vi "FileController.vi"() -> ()   [LabVIEW 2018]
panel:
  in  "Overdrive":bool
  in  "New file":bool
  in  "Pause DAQ":bool
  in  "Record":bool
  in  "Valve Log Name":string
  in  "Load Cell Log Name":string
  in  "Sensor Log Name":string
  in  "Log Folder":path
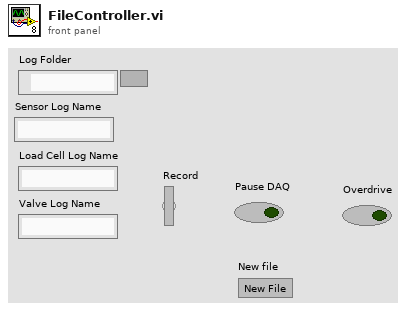
[diagram p1: front panel]
types:
  T1 = cluster{"SensorRecState":refnum<notifier>, "LoadCellRecState":refnum<notifier>, "ValveRecState":refnum<notifier>}
  T2 = enum16{"Normal", "Overdrive", "Ready for Overdrive End", "Ready for new file", "New file"}
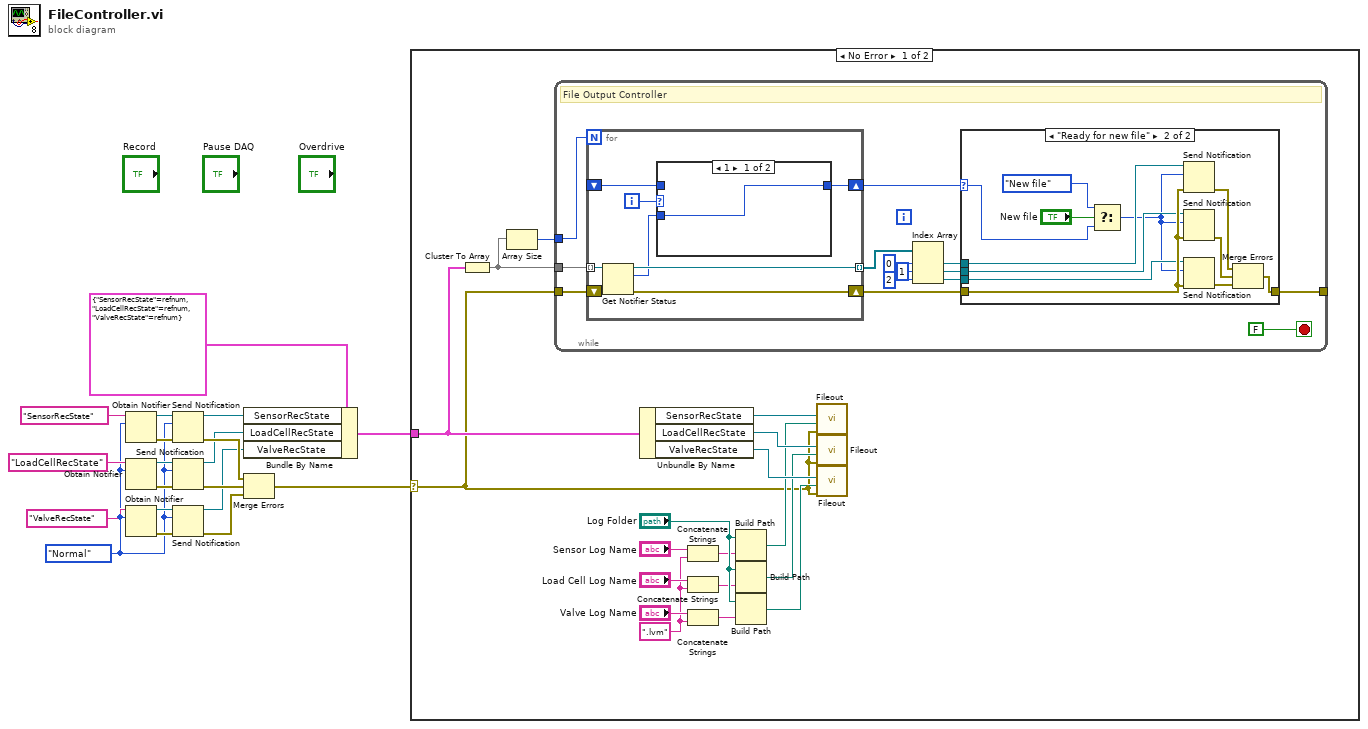
[diagram p0: block diagram]
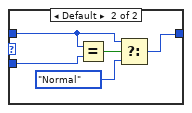
[diagram p3: hidden frame]
diagram:
  w1 = T2."Normal" ("RecState")
  n1 = Obtain Notifier(name (unnamed)="SensorRecState", notification data type=w1) -> (notifier out=w8:refnum<notifier>, error out=w9:errorcluster)  [unwired: 2 in, 1 out]
  n2 = Obtain Notifier(name (unnamed)="LoadCellRecState", notification data type=w1) -> (notifier out=w10:refnum<notifier>, error out=w11:errorcluster)  [unwired: 2 in, 1 out]
  n3 = Obtain Notifier(name (unnamed)="ValveRecState", notification data type=w1) -> (notifier out=w12:refnum<notifier>, error out=w13:errorcluster)  [unwired: 2 in, 1 out]
  n4 = Send Notification(notification=w1, notifier=w8, error in (no error)=w9) -> (notifier out=w7:refnum<notifier>, error out=w6:errorcluster)
  n5 = Send Notification(notification=w1, notifier=w10, error in (no error)=w11) -> (notifier out=w4:refnum<notifier>, error out=w5:errorcluster)
  n6 = Send Notification(notification=w1, notifier=w12, error in (no error)=w13) -> (notifier out=w3:refnum<notifier>, error out=w2:errorcluster)
  n7 = Bundle By Name(cluster=T1 {"SensorRecState"=refnum, "LoadCellRecState"=refnum, "ValveRecState"=refnum} ("input cluster"), "SensorRecState"=w7, "LoadCellRecState"=w4, "ValveRecState"=w3) -> (w15:T1)
  n8 = Merge Errors(w6, w5, w2) -> (w16:errorcluster)
  n9 = case shown="No Error" w16 {
    selector: w16 -> [w20 _]
    tunnel: w15 -> [w27 _]
    frame No Error {
      w32 = ".lvm"
      n10 = Cluster To Array(cluster=w27) -> (array=w37:refnum<notifier>[])
      n11 = Array Size(array=w37) -> (size(s)=w36:i32)
      n12 = while {
        tunnel: w37 -> [w50]
        tunnel: w36 -> [w51]
        tunnel: w20 -> [w49]
        tunnel: [w38] -> _
        stop <- FALSE stop-if-true
        # "File Output Controller"
        n13 = for {
          N: w51 -> [_]
          tunnel: w50 -> [w72] mode=indexing
          shift-right: [w70] -> w43
          shift-left: w49 -> [w71]
          shift-right: [w66] -> w44
          shift-left: _ -> [w68]
          tunnel: [w67] -> w48 mode=indexing
          i -> [w69]
          n14 = Get Notifier Status(notifier=w72, error in (no error)=w71) -> (notifier out=w67:refnum<notifier>, current notification=w65:T2, error out=w70:errorcluster)  [unwired: 2 out]
          n15 = case shown="1" w69 {
            tunnel: w65 -> [w73 w78]
            tunnel: [w73 w74] -> w66
            tunnel: w68 -> [_ w76]
            frame 1 {
            }
            frame Default {
              n16 = Equal?(x=w76, y=w78) -> (x = y?=w77:bool)
              n17 = Select(t=w76, s=w77, f=T2."Normal" ("RecState")) -> (s? t:f=w74:T2)
            }
          }
        }
        n18 = Index Array(array=w48, index #1=0 ("index"), index #2=1 ("index"), index #3=2 ("index")) -> (element #1=w39:refnum<notifier>, element #2=w40:refnum<notifier>, element #3=w41:refnum<notifier>)
        n19 = case shown="\"Ready for new file\"" w44 {
          selector: w44 -> [_ w60]
          tunnel: w43 -> [w52 w64]
          tunnel: w41 -> [_ w63]
          tunnel: w40 -> [_ w62]
          tunnel: w39 -> [_ w61]
          tunnel: [w52 w53] -> w38
          frame "Normal", Default {
          }
          frame "Ready for new file" {
            n20 = Select(t=T2."New file" ("RecState"), s="New file", f=w60) -> (s? t:f=w57:T2)
            n21 = Send Notification(notification=w57, notifier=w61, error in (no error)=w64) -> (error out=w54:errorcluster)  [unwired: 1 out]
            n22 = Send Notification(notification=w57, notifier=w62, error in (no error)=w64) -> (error out=w55:errorcluster)  [unwired: 1 out]
            n23 = Send Notification(notification=w57, notifier=w63, error in (no error)=w64) -> (error out=w56:errorcluster)  [unwired: 1 out]
            n24 = Merge Errors(w54, w55, w56) -> (w53:errorcluster)
          }
        }
      }
      n25 = Unbundle By Name(w27) -> ("SensorRecState"=w26:refnum<notifier>, "LoadCellRecState"=w25:refnum<notifier>, "ValveRecState"=w24:refnum<notifier>)
      n26 = Concatenate Strings("Sensor Log Name", w32) -> (w30:string)
      n27 = Concatenate Strings("Load Cell Log Name", w32) -> (w29:string)
      n28 = Concatenate Strings("Valve Log Name", w32) -> (w28:string)
      n29 = Build Path(base path="Log Folder", name or relative path=w30) -> (appended path=w23:path)
      n30 = Build Path(base path="Log Folder", name or relative path=w29) -> (appended path=w22:path)
      n31 = Build Path(base path="Log Folder", name or relative path=w28) -> (appended path=w21:path)
      n32 = call "Fileout.vi"("error in (no error)"=w20, "Filepath"=w23, "RecState"=w26) -> ()  [unwired: 8 in, 1 out]
      n33 = call "Fileout.vi"("error in (no error)"=w20, "Filepath"=w22, "RecState"=w25) -> ()  [unwired: 8 in, 1 out]
      n34 = call "Fileout.vi"("error in (no error)"=w20, "Filepath"=w21, "RecState"=w24) -> ()  [unwired: 8 in, 1 out]
    }
    frame Error {
    }
  }
